vi "ArmGoToPosition.vi"(0 "RobotConfig":T15={"Motors"={"DriveRightPrimary"={"CAN Address"=3, "Invert"=FALSE, "InvertSensor"=FALSE, "Unit Conversion Factor"=0.0, "Brake Mode"=enum."Override to Brake", "Reverse Limt Switch Mode"=enum."Normally Closed", "Forward Limt Swith Mode"=enum."Normally Closed", "PWM Channel"=enum."Invalid", "Motor Controller Type"=enum."Talon SRX", "Peak Current (A)"=0, "Continuous Current (A)"=0, "Peak Duration (ms)"=0, "Current Limit Enable"=FALSE}, "DriveRightSecondary"={"CAN Address"=2, "Invert"=FALSE, "InvertSensor"=FALSE, "Unit Conversion Factor"=0.0, "Brake Mode"=enum."Override to Brake", "Reverse Limt Switch Mode"=enum."Normally Closed", "Forward Limt Swith Mode"=enum."Normally Closed", "PWM Channel"=enum."Invalid", "Motor Controller Type"=enum."Talon SRX", "Peak Current (A)"=0, "Continuous Current (A)"=0, "Peak Duration (ms)"=0, "Current Limit Enable"=FALSE}, "DriveLeftPrimary"={"CAN Address"=1, "Invert"=FALSE, "InvertSensor"=FALSE, "Unit Conversion Factor"=0.0, "Brake Mode"=enum."Override to Brake", "Reverse Limt Switch Mode"=enum."Normally Closed", "Forward Limt Swith Mode"=enum."Normally Closed", "PWM Channel"=enum."Invalid", "Motor Controller Type"=enum."Talon SRX", "Peak Current (A)"=0, "Continuous Current (A)"=0, "Peak Duration (ms)"=0, "Current Limit Enable"=FALSE}, "DriveLeftSecondary"={"CAN Address"=4, "Invert"=FALSE, "InvertSensor"=FALSE, "Unit Conversion Factor"=0.0, "Brake Mode"=enum."Override to Brake", "Reverse Limt Switch Mode"=enum."Normally Closed", "Forward Limt Swith Mode"=enum."Normally Closed", "PWM Channel"=enum."Invalid", "Motor Controller Type"=enum."Talon SRX", "Peak Current (A)"=0, "Continuous Current (A)"=0, "Peak Duration (ms)"=0, "Current Limit Enable"=FALSE}, "RearClimb"={"CAN Address"=8, "Invert"=FALSE, "InvertSensor"=FALSE, "Unit Conversion Factor"=0.0, "Brake Mode"=enum."Override to Brake", "Reverse Limt Switch Mode"=enum."Normally Closed", "Forward Limt Swith Mode"=enum."Normally Closed", "PWM Channel"=enum."Invalid", "Motor Controller Type"=enum."Talon SRX", "Peak Current (A)"=0, "Continuous Current (A)"=0, "Peak Duration (ms)"=0, "Current Limit Enable"=FALSE}, "Front Climb"={"CAN Address"=7, "Invert"=FALSE, "InvertSensor"=FALSE, "Unit Conversion Factor"=0.0, "Brake Mode"=enum."Override to Brake", "Reverse Limt Switch Mode"=enum."Normally Closed", "Forward Limt Swith Mode"=enum."Normally Closed", "PWM Channel"=enum."Invalid", "Motor Controller Type"=enum."Talon SRX", "Peak Current (A)"=0, "Continuous Current (A)"=0, "Peak Duration (ms)"=0, "Current Limit Enable"=FALSE}, "Climb Drive"={"CAN Address"=5, "Invert"=FALSE, "InvertSensor"=FALSE, "Unit Conversion Factor"=0.0, "Brake Mode"=enum."Override to Brake", "Reverse Limt Switch Mode"=enum."Normally Closed", "Forward Limt Swith Mode"=enum."Normally Closed", "PWM Channel"=enum."Invalid", "Motor Controller Type"=enum."Talon SRX", "Peak Current (A)"=0, "Continuous Current (A)"=0, "Peak Duration (ms)"=0, "Current Limit Enable"=FALSE}, "Shoulder1"={"CAN Address"=6, "Invert"=FALSE, "InvertSensor"=FALSE, "Unit Conversion Factor"=0.0, "Brake Mode"=enum."Override to Brake", "Reverse Limt Switch Mode"=enum."Normally Closed", "Forward Limt Swith Mode"=enum."Normally Closed", "PWM Channel"=enum."Invalid", "Motor Controller Type"=enum."Talon SRX", "Peak Current (A)"=0, "Continuous Current (A)"=0, "Peak Duration (ms)"=0, "Current Limit Enable"=FALSE}, "Shoulder2"={"CAN Address"=9, "Invert"=FALSE, "InvertSensor"=FALSE, "Unit Conversion Factor"=0.0, "Brake Mode"=enum."Override to Brake", "Reverse Limt Switch Mode"=enum."Normally Closed", "Forward Limt Swith Mode"=enum."Normally Closed", "PWM Channel"=enum."Invalid", "Motor Controller Type"=enum."Talon SRX", "Peak Current (A)"=0, "Continuous Current (A)"=0, "Peak Duration (ms)"=0, "Current Limit Enable"=FALSE}, "Wrist"={"CAN Address"=10, "Invert"=FALSE, "InvertSensor"=FALSE, "Unit Conversion Factor"=0.0, "Brake Mode"=enum."Override to Brake", "Reverse Limt Switch Mode"=enum."Disabled", "Forward Limt Swith Mode"=enum."Disabled", "PWM Channel"=enum."Invalid", "Motor Controller Type"=enum."Talon SRX", "Peak Current (A)"=0, "Continuous Current (A)"=0, "Peak Duration (ms)"=0, "Current Limit Enable"=FALSE}, "Extension"={"CAN Address"=11, "Invert"=FALSE, "InvertSensor"=FALSE, "Unit Conversion Factor"=0.0, "Brake Mode"=enum."Override to Brake", "Reverse Limt Switch Mode"=enum."Disabled", "Forward Limt Swith Mode"=enum."Disabled", "PWM Channel"=enum."Invalid", "Motor Controller Type"=enum."Talon SRX", "Peak Current (A)"=0, "Continuous Current (A)"=0, "Peak Duration (ms)"=0, "Current Limit Enable"=FALSE}, "CargoIntake"={"CAN Address"=0, "Invert"=FALSE, "InvertSensor"=FALSE, "Unit Conversion Factor"=1.0, "Brake Mode"=enum."Override to Brake", "Reverse Limt Switch Mode"=enum."Disabled", "Forward Limt Swith Mode"=enum."Normally Open", "PWM Channel"=enum."PWM 8", "Motor Controller Type"=enum."Talon SR", "Peak Current (A)"=0, "Continuous Current (A)"=0, "Peak Duration (ms)"=0, "Current Limit Enable"=FALSE}, "Intake2"={"CAN Address"=10, "Invert"=FALSE, "InvertSensor"=TRUE, "Unit Conversion Factor"=0.0, "Brake Mode"=enum."Override to Brake", "Reverse Limt Switch Mode"=enum."Normally Open", "Forward Limt Swith Mode"=enum."Normally Open", "PWM Channel"=enum."PWM 0", "Motor Controller Type"=enum."Disabled", "Peak Current (A)"=0, "Continuous Current (A)"=0, "Peak Duration (ms)"=0, "Current Limit Enable"=FALSE}}, "Sensors"={"IMU"={"Yaw Axis"=enum."Z", "SPI Bus"=enum."SPI MXP", "AHRS Algorithm"=enum."Complementary", "Calibration Time (s)"=3.0, "Calibrate On Open"=TRUE}, "HomingButton"={"DIOChannel"=enum."DIO 0", "Active Low"=FALSE}, "HomingLED_Green"={"DIOChannel"=enum."DIO 0", "Active Low"=FALSE}, "HomingLED_Yellow"={"DIOChannel"=enum."DIO 0", "Active Low"=FALSE}, "HomingLED_Red"={"DIOChannel"=enum."DIO 0", "Active Low"=FALSE}}, "PID"={"FrontClimb"={"P"=0.0, "I"=0.0, "D"=0.0, "F"=0.0, "IZone"=0.0}, "RearClimb"={"P"=0.0, "I"=0.0, "D"=0.0, "F"=0.0, "IZone"=0.0}, "ArmShoulder"={"P"=0.0, "I"=0.0, "D"=0.0, "F"=0.0, "IZone"=0.0}, "ArmExtend"={"P"=0.0, "I"=0.0, "D"=0.0, "F"=0.0, "IZone"=0.0}, "ArmWrist"={"P"=0.0, "I"=0.0, "D"=0.0, "F"=0.0, "IZone"=0.0}}, "Solenoids"={" Shifter"={"SolenoidChannel"=enum."Solenoid 3", "Invert"=FALSE}, "Hatch Grip"={"SolenoidChannel"=enum."Solenoid 0", "Invert"=FALSE}, "Hatch Extend"={"SolenoidChannel"=enum."Solenoid 1", "Invert"=FALSE}, "Manipulator Slide"={"SolenoidChannel"=enum."Solenoid 2", "Invert"=FALSE}, "Hatch Floor Intake"={"SolenoidChannel"=enum."Solenoid 0", "Invert"=FALSE}}, "Enable Compressor"=TRUE, "MotionMagic"={"FrontClimbExtend"={"CruiseVelocity"=0, "Acceleration"=0}, "RearClimbExtend"={"CruiseVelocity"=0, "Acceleration"=0}, "FrontClimbRetract"={"CruiseVelocity"=0, "Acceleration"=0}, "RearClimbRetract"={"CruiseVelocity"=0, "Acceleration"=0}}, "RobotDimensions"={"Length (in)"=0.0, "Shoulder Height (in)"=0.0, "Frame Height (in)"=0.0, "Arm Center to Front of Robot (in)"=0.0, "Arm Min Extension (in)"=0.0, "Arm Max Extension (in)"=0.0, "Cargo Intake Loop Length (in)"=0.0, "Cargo Intake Loop Width (in)"=0.0, "Cargo Intake Loop Offset (in)"=0.0, "Cargo Intake Loop Angle (rad)"=0.0}, "Arm Home Position"={"Radius (in)"=0.0, "ShoulderAngle (rad)"=0.0, "WristAngle (rad)"=0.0}, "Climb Home Position"={"Back Climb"=0.0, "Front Climb"=0.0}, "Climb Positions"={"Retract"=0.0, "Level 2"=0.0, "Level 3"=0.0}}, 1 "ArmPlanRequest":T10={"Destination"=enum."Forward Cargo Feeder Station", "Preview"=FALSE, "Start"=enum."Forward Cargo Feeder Station", "Fixed Start"=FALSE}, 2 "Arm min Extension (in)":dbl, 3 "Arm max Extension (in)":dbl, 4 "Game Piece Position":T32, 5 "Avoidance Polygon":T30, 6 "RobotMotors":T4={"DriveRightPrimary"={"DeviceStatus"={"status"=FALSE, "code"=0, "source"=""}, "Type"=enum."PWM", "PWM"={"PWM Channel"=enum."PWM 1", "DeadBand"={"Name"="", "maxPositivePwm"=0, "minPositivePwm"=0, "centerPwm"=0, "maxNegativePwm"=0, "minNegativePwm"=0, "angularRange"=0}}, "CAN"={"Device Number"=0, "SetOutput VI Ref"=variant(enum8{"Percent VBus", "Current", "Speed", "Position", "Voltage"} enum."Percent VBus"), "GetOutput VI Ref"=variant(refnum<k1> refnum), "Enable VI Ref"=variant(dbl 12.0), "Disable VI Ref"=variant(enum8{"Percent VBus", "Speed", "Position", "Slave", "Unchanged / Invalid", "Voltage Compensation", "Current", "Motion Profile"} enum."Percent VBus"), "Data"=variant}, "Invert"=FALSE, "DIO PWM"={"PWM \"Enable\" Channel"=enum."Invalid", "DIOChannel"=enum."Invalid", "PWM Rate"=0.0}}, "DriveRightSecondary"={"DeviceStatus"={"status"=FALSE, "code"=0, "source"=""}, "Type"=enum."PWM", "PWM"={"PWM Channel"=enum."PWM 1", "DeadBand"={"Name"="", "maxPositivePwm"=0, "minPositivePwm"=0, "centerPwm"=0, "maxNegativePwm"=0, "minNegativePwm"=0, "angularRange"=0}}, "CAN"={"Device Number"=0, "SetOutput VI Ref"=variant(enum8{"Percent VBus", "Current", "Speed", "Position", "Voltage"} enum."Percent VBus"), "GetOutput VI Ref"=variant(refnum<k1> refnum), "Enable VI Ref"=variant(dbl 12.0), "Disable VI Ref"=variant(enum8{"Percent VBus", "Speed", "Position", "Slave", "Unchanged / Invalid", "Voltage Compensation", "Current", "Motion Profile"} enum."Percent VBus"), "Data"=variant}, "Invert"=FALSE, "DIO PWM"={"PWM \"Enable\" Channel"=enum."Invalid", "DIOChannel"=enum."Invalid", "PWM Rate"=0.0}}, "DriveLeftPrimary"={"DeviceStatus"={"status"=FALSE, "code"=0, "source"=""}, "Type"=enum."PWM", "PWM"={"PWM Channel"=enum."PWM 1", "DeadBand"={"Name"="", "maxPositivePwm"=0, "minPositivePwm"=0, "centerPwm"=0, "maxNegativePwm"=0, "minNegativePwm"=0, "angularRange"=0}}, "CAN"={"Device Number"=0, "SetOutput VI Ref"=variant(enum8{"Percent VBus", "Current", "Speed", "Position", "Voltage"} enum."Percent VBus"), "GetOutput VI Ref"=variant(refnum<k1> refnum), "Enable VI Ref"=variant(dbl 12.0), "Disable VI Ref"=variant(enum8{"Percent VBus", "Speed", "Position", "Slave", "Unchanged / Invalid", "Voltage Compensation", "Current", "Motion Profile"} enum."Percent VBus"), "Data"=variant}, "Invert"=FALSE, "DIO PWM"={"PWM \"Enable\" Channel"=enum."Invalid", "DIOChannel"=enum."Invalid", "PWM Rate"=0.0}}, "DriveLeftSecondary"={"DeviceStatus"={"status"=FALSE, "code"=0, "source"=""}, "Type"=enum."PWM", "PWM"={"PWM Channel"=enum."PWM 1", "DeadBand"={"Name"="", "maxPositivePwm"=0, "minPositivePwm"=0, "centerPwm"=0, "maxNegativePwm"=0, "minNegativePwm"=0, "angularRange"=0}}, "CAN"={"Device Number"=0, "SetOutput VI Ref"=variant(enum8{"Percent VBus", "Current", "Speed", "Position", "Voltage"} enum."Percent VBus"), "GetOutput VI Ref"=variant(refnum<k1> refnum), "Enable VI Ref"=variant(dbl 12.0), "Disable VI Ref"=variant(enum8{"Percent VBus", "Speed", "Position", "Slave", "Unchanged / Invalid", "Voltage Compensation", "Current", "Motion Profile"} enum."Percent VBus"), "Data"=variant}, "Invert"=FALSE, "DIO PWM"={"PWM \"Enable\" Channel"=enum."Invalid", "DIOChannel"=enum."Invalid", "PWM Rate"=0.0}}, " RearClimb"={"DeviceStatus"={"status"=FALSE, "code"=0, "source"=""}, "Type"=enum."PWM", "PWM"={"PWM Channel"=enum."PWM 1", "DeadBand"={"Name"="", "maxPositivePwm"=0, "minPositivePwm"=0, "centerPwm"=0, "maxNegativePwm"=0, "minNegativePwm"=0, "angularRange"=0}}, "CAN"={"Device Number"=0, "SetOutput VI Ref"=variant(enum8{"Percent VBus", "Current", "Speed", "Position", "Voltage"} enum."Percent VBus"), "GetOutput VI Ref"=variant(refnum<k1> refnum), "Enable VI Ref"=variant(dbl 12.0), "Disable VI Ref"=variant(enum8{"Percent VBus", "Speed", "Position", "Slave", "Unchanged / Invalid", "Voltage Compensation", "Current", "Motion Profile"} enum."Percent VBus"), "Data"=variant}, "Invert"=FALSE, "DIO PWM"={"PWM \"Enable\" Channel"=enum."Invalid", "DIOChannel"=enum."Invalid", "PWM Rate"=0.0}}, "FrontClimb"={"DeviceStatus"={"status"=FALSE, "code"=0, "source"=""}, "Type"=enum."PWM", "PWM"={"PWM Channel"=enum."PWM 1", "DeadBand"={"Name"="", "maxPositivePwm"=0, "minPositivePwm"=0, "centerPwm"=0, "maxNegativePwm"=0, "minNegativePwm"=0, "angularRange"=0}}, "CAN"={"Device Number"=0, "SetOutput VI Ref"=variant(enum8{"Percent VBus", "Current", "Speed", "Position", "Voltage"} enum."Percent VBus"), "GetOutput VI Ref"=variant(refnum<k1> refnum), "Enable VI Ref"=variant(dbl 12.0), "Disable VI Ref"=variant(enum8{"Percent VBus", "Speed", "Position", "Slave", "Unchanged / Invalid", "Voltage Compensation", "Current", "Motion Profile"} enum."Percent VBus"), "Data"=variant}, "Invert"=FALSE, "DIO PWM"={"PWM \"Enable\" Channel"=enum."Invalid", "DIOChannel"=enum."Invalid", "PWM Rate"=0.0}}, "ClimbDrive"={"DeviceStatus"={"status"=FALSE, "code"=0, "source"=""}, "Type"=enum."PWM", "PWM"={"PWM Channel"=enum."PWM 1", "DeadBand"={"Name"="", "maxPositivePwm"=0, "minPositivePwm"=0, "centerPwm"=0, "maxNegativePwm"=0, "minNegativePwm"=0, "angularRange"=0}}, "CAN"={"Device Number"=0, "SetOutput VI Ref"=variant(enum8{"Percent VBus", "Current", "Speed", "Position", "Voltage"} enum."Percent VBus"), "GetOutput VI Ref"=variant(refnum<k1> refnum), "Enable VI Ref"=variant(dbl 12.0), "Disable VI Ref"=variant(enum8{"Percent VBus", "Speed", "Position", "Slave", "Unchanged / Invalid", "Voltage Compensation", "Current", "Motion Profile"} enum."Percent VBus"), "Data"=variant}, "Invert"=FALSE, "DIO PWM"={"PWM \"Enable\" Channel"=enum."Invalid", "DIOChannel"=enum."Invalid", "PWM Rate"=0.0}}, "Shoulder2"={"DeviceStatus"={"status"=FALSE, "code"=0, "source"=""}, "Type"=enum."PWM", "PWM"={"PWM Channel"=enum."PWM 1", "DeadBand"={"Name"="", "maxPositivePwm"=0, "minPositivePwm"=0, "centerPwm"=0, "maxNegativePwm"=0, "minNegativePwm"=0, "angularRange"=0}}, "CAN"={"Device Number"=0, "SetOutput VI Ref"=variant(enum8{"Percent VBus", "Current", "Speed", "Position", "Voltage"} enum."Percent VBus"), "GetOutput VI Ref"=variant(refnum<k1> refnum), "Enable VI Ref"=variant(dbl 12.0), "Disable VI Ref"=variant(enum8{"Percent VBus", "Speed", "Position", "Slave", "Unchanged / Invalid", "Voltage Compensation", "Current", "Motion Profile"} enum."Percent VBus"), "Data"=variant}, "Invert"=FALSE, "DIO PWM"={"PWM \"Enable\" Channel"=enum."Invalid", "DIOChannel"=enum."Invalid", "PWM Rate"=0.0}}, "Shoulder1 "={"DeviceStatus"={"status"=FALSE, "code"=0, "source"=""}, "Type"=enum."PWM", "PWM"={"PWM Channel"=enum."PWM 1", "DeadBand"={"Name"="", "maxPositivePwm"=0, "minPositivePwm"=0, "centerPwm"=0, "maxNegativePwm"=0, "minNegativePwm"=0, "angularRange"=0}}, "CAN"={"Device Number"=0, "SetOutput VI Ref"=variant(enum8{"Percent VBus", "Current", "Speed", "Position", "Voltage"} enum."Percent VBus"), "GetOutput VI Ref"=variant(refnum<k1> refnum), "Enable VI Ref"=variant(dbl 12.0), "Disable VI Ref"=variant(enum8{"Percent VBus", "Speed", "Position", "Slave", "Unchanged / Invalid", "Voltage Compensation", "Current", "Motion Profile"} enum."Percent VBus"), "Data"=variant}, "Invert"=FALSE, "DIO PWM"={"PWM \"Enable\" Channel"=enum."Invalid", "DIOChannel"=enum."Invalid", "PWM Rate"=0.0}}, "Wrist"={"DeviceStatus"={"status"=FALSE, "code"=0, "source"=""}, "Type"=enum."PWM", "PWM"={"PWM Channel"=enum."PWM 1", "DeadBand"={"Name"="", "maxPositivePwm"=0, "minPositivePwm"=0, "centerPwm"=0, "maxNegativePwm"=0, "minNegativePwm"=0, "angularRange"=0}}, "CAN"={"Device Number"=0, "SetOutput VI Ref"=variant(enum8{"Percent VBus", "Current", "Speed", "Position", "Voltage"} enum."Percent VBus"), "GetOutput VI Ref"=variant(refnum<k1> refnum), "Enable VI Ref"=variant(dbl 12.0), "Disable VI Ref"=variant(enum8{"Percent VBus", "Speed", "Position", "Slave", "Unchanged / Invalid", "Voltage Compensation", "Current", "Motion Profile"} enum."Percent VBus"), "Data"=variant}, "Invert"=FALSE, "DIO PWM"={"PWM \"Enable\" Channel"=enum."Invalid", "DIOChannel"=enum."Invalid", "PWM Rate"=0.0}}, "Extension"={"DeviceStatus"={"status"=FALSE, "code"=0, "source"=""}, "Type"=enum."PWM", "PWM"={"PWM Channel"=enum."PWM 1", "DeadBand"={"Name"="", "maxPositivePwm"=0, "minPositivePwm"=0, "centerPwm"=0, "maxNegativePwm"=0, "minNegativePwm"=0, "angularRange"=0}}, "CAN"={"Device Number"=0, "SetOutput VI Ref"=variant(enum8{"Percent VBus", "Current", "Speed", "Position", "Voltage"} enum."Percent VBus"), "GetOutput VI Ref"=variant(refnum<k1> refnum), "Enable VI Ref"=variant(dbl 12.0), "Disable VI Ref"=variant(enum8{"Percent VBus", "Speed", "Position", "Slave", "Unchanged / Invalid", "Voltage Compensation", "Current", "Motion Profile"} enum."Percent VBus"), "Data"=variant}, "Invert"=FALSE, "DIO PWM"={"PWM \"Enable\" Channel"=enum."Invalid", "DIOChannel"=enum."Invalid", "PWM Rate"=0.0}}, "CargoIntake"={"DeviceStatus"={"status"=FALSE, "code"=0, "source"=""}, "Type"=enum."PWM", "PWM"={"PWM Channel"=enum."PWM 1", "DeadBand"={"Name"="", "maxPositivePwm"=0, "minPositivePwm"=0, "centerPwm"=0, "maxNegativePwm"=0, "minNegativePwm"=0, "angularRange"=0}}, "CAN"={"Device Number"=0, "SetOutput VI Ref"=variant(enum8{"Percent VBus", "Current", "Speed", "Position", "Voltage"} enum."Percent VBus"), "GetOutput VI Ref"=variant(refnum<k1> refnum), "Enable VI Ref"=variant(dbl 12.0), "Disable VI Ref"=variant(enum8{"Percent VBus", "Speed", "Position", "Slave", "Unchanged / Invalid", "Voltage Compensation", "Current", "Motion Profile"} enum."Percent VBus"), "Data"=variant}, "Invert"=FALSE, "DIO PWM"={"PWM \"Enable\" Channel"=enum."Invalid", "DIOChannel"=enum."Invalid", "PWM Rate"=0.0}}, "Intake2"={"DeviceStatus"={"status"=FALSE, "code"=0, "source"=""}, "Type"=enum."PWM", "PWM"={"PWM Channel"=enum."PWM 1", "DeadBand"={"Name"="", "maxPositivePwm"=0, "minPositivePwm"=0, "centerPwm"=0, "maxNegativePwm"=0, "minNegativePwm"=0, "angularRange"=0}}, "CAN"={"Device Number"=0, "SetOutput VI Ref"=variant(enum8{"Percent VBus", "Current", "Speed", "Position", "Voltage"} enum."Percent VBus"), "GetOutput VI Ref"=variant(refnum<k1> refnum), "Enable VI Ref"=variant(dbl 12.0), "Disable VI Ref"=variant(enum8{"Percent VBus", "Speed", "Position", "Slave", "Unchanged / Invalid", "Voltage Compensation", "Current", "Motion Profile"} enum."Percent VBus"), "Data"=variant}, "Invert"=FALSE, "DIO PWM"={"PWM \"Enable\" Channel"=enum."Invalid", "DIOChannel"=enum."Invalid", "PWM Rate"=0.0}}}, 7 "MotionProfileGeneratorParameters":T29={"Trajectory Point Interval (ms)"=10, "Maximum Travel Speed (units/s)"=0.0, "Velocity Ramp Time (ms)"=0.0, "Acceleration Ramp Time (ms)"=1.0} {"Acceleration Ramp Time (ms)" min=1.0; "Velocity Ramp Time (ms)" min=1.0; "Maximum Travel Speed (units/s)" min=0.0; "Trajectory Point Interval (ms)" items=["TrajectoryDuration_0ms"=0, "TrajectoryDuration_5ms"=5, "TrajectoryDuration_10ms"=10, "TrajectoryDuration_20ms"=20, "TrajectoryDuration_30ms"=30, "TrajectoryDuration_40ms"=40, "TrajectoryDuration_50ms"=50, "TrajectoryDuration_100ms"=100]}, 8 "Arm Pass Through Params":T2, 9 "RobotDimensions":T3, 10 "TestMode":bool, 11 "Test_ArmAbsolutePose":T1) -> (14 "ArmPlanResponse":T12 {"WristTrajectory"."Time (ms)" items=["TrajectoryDuration_0ms"=0, "TrajectoryDuration_5ms"=5, "TrajectoryDuration_10ms"=10, "TrajectoryDuration_20ms"=20, "TrajectoryDuration_30ms"=30, "TrajectoryDuration_40ms"=40, "TrajectoryDuration_50ms"=50, "TrajectoryDuration_100ms"=100]; "ExtendTrajectory"."Time (ms)" items=["TrajectoryDuration_0ms"=0, "TrajectoryDuration_5ms"=5, "TrajectoryDuration_10ms"=10, "TrajectoryDuration_20ms"=20, "TrajectoryDuration_30ms"=30, "TrajectoryDuration_40ms"=40, "TrajectoryDuration_50ms"=50, "TrajectoryDuration_100ms"=100]; "ShoulderTrajectory"."Time (ms)" items=["TrajectoryDuration_0ms"=0, "TrajectoryDuration_5ms"=5, "TrajectoryDuration_10ms"=10, "TrajectoryDuration_20ms"=20, "TrajectoryDuration_30ms"=30, "TrajectoryDuration_40ms"=40, "TrajectoryDuration_50ms"=50, "TrajectoryDuration_100ms"=100]})   [LabVIEW 2018]
uses:
  TypeDefs/GamePiecePosition.ctl
  TypeDefs/ArmPositions.ctl
  TypeDefs/ArmAbsolutePosition.ctl
  ArgosLib/Path Planning/TypeDefs/Polygon2D.ctl
  ArgosLib/Path Planning/TypeDefs/Point2D.ctl
  ArgosLib/MotionProfiling/TypeDefs/MotionProfileGeneratorParams.ctl
  <vilib>/Rock Robotics/WPI/ThirdParty/Phoenix-LabVIEW/Motor Controller/Controls/CTRE_Phoenix_MotorControl_TrajectoryPointTimeDur.ctl
  TypeDefs/ConfigComponents/Config_Robot.ctl
  ArgosLib/Config/ConfigComponents/TypeDefs/Config_Motor.ctl
  <vilib>/Rock Robotics/WPI/ThirdParty/Phoenix-LabVIEW/Motor Controller/Controls/CTRE_Phoenix_MotorControl_NeutralMode.ctl
  <vilib>/Rock Robotics/WPI/ThirdParty/Phoenix-LabVIEW/Motor Controller/Controls/CTRE_Phoenix_MotorControl_LimitSwitchNormal.ctl
  <vilib>/Rock Robotics/SystemInterfaces/DIO/FPGA_DIOPWMChannel.ctl
  ArgosLib/Config/ConfigComponents/TypeDefs/Config_MotorCtrlType.ctl
  ArgosLib/Config/ConfigComponents/TypeDefs/Config_IMU.ctl
  <vilib>/Rock Robotics/SystemInterfaces/spilib/spi_bus.ctl
  ArgosLib/Config/ConfigComponents/TypeDefs/Config_DigitalIO.ctl
  <vilib>/Rock Robotics/SystemInterfaces/DIO/FPGA_DIOChannel.ctl
  ArgosLib/Config/ConfigComponents/TypeDefs/Config_PIDParams.ctl
  ArgosLib/Config/ConfigComponents/TypeDefs/Config_SingleSolenoid.ctl
  <vilib>/Rock Robotics/WPI/Solenoid/WPI_SolenoidChannel.ctl
  ArgosLib/Config/ConfigComponents/TypeDefs/Config_MotionMagicParams.ctl
  TypeDefs/ConfigComponents/Config_Dimensions.ctl
  TypeDefs/ArmCoordinate.ctl
  Climber/TypeDefs/ClimberPositionHeights.ctl
  TypeDefs/ArmPlanResponse.ctl
  ArgosLib/MotionProfiling/TypeDefs/TrajectoryPoint.ctl
  TypeDefs/ArmPlanRequest.ctl
  TypeDefs/ArmTargetPosition.ctl
  TypeDefs/RobotComponents/RobotMotors.ctl
  <vilib>/Rock Robotics/WPI/MotorControl/WPI_MotorControlDeviceRef.ctl
  <vilib>/Rock Robotics/WPI/MotorControl/WPI_MotorControlType.ctl
  <vilib>/Rock Robotics/WPI/PWM/WPI_PWMDeadband.ctl
  TypeDefs/ArmPassThroughParams.ctl
  <vilib>/Playing With Fusion Inc/Playing With Fusion Lib for FRC/PWF_Venom_LabVIEW/Public/PwF_Venom_GetPosition.vi
  <vilib>/Rock Robotics/WPI/ThirdParty/Phoenix-LabVIEW/Motor Controller/Get/CTRE_Phoenix_MotorController_GetSelectedSensorData.vi
  ArgosLib/ArgosLib.lvlib
  <vilib>/Playing With Fusion Inc/Playing With Fusion Lib for FRC/PWF_Venom_LabVIEW/PwF_Venom.lvlib
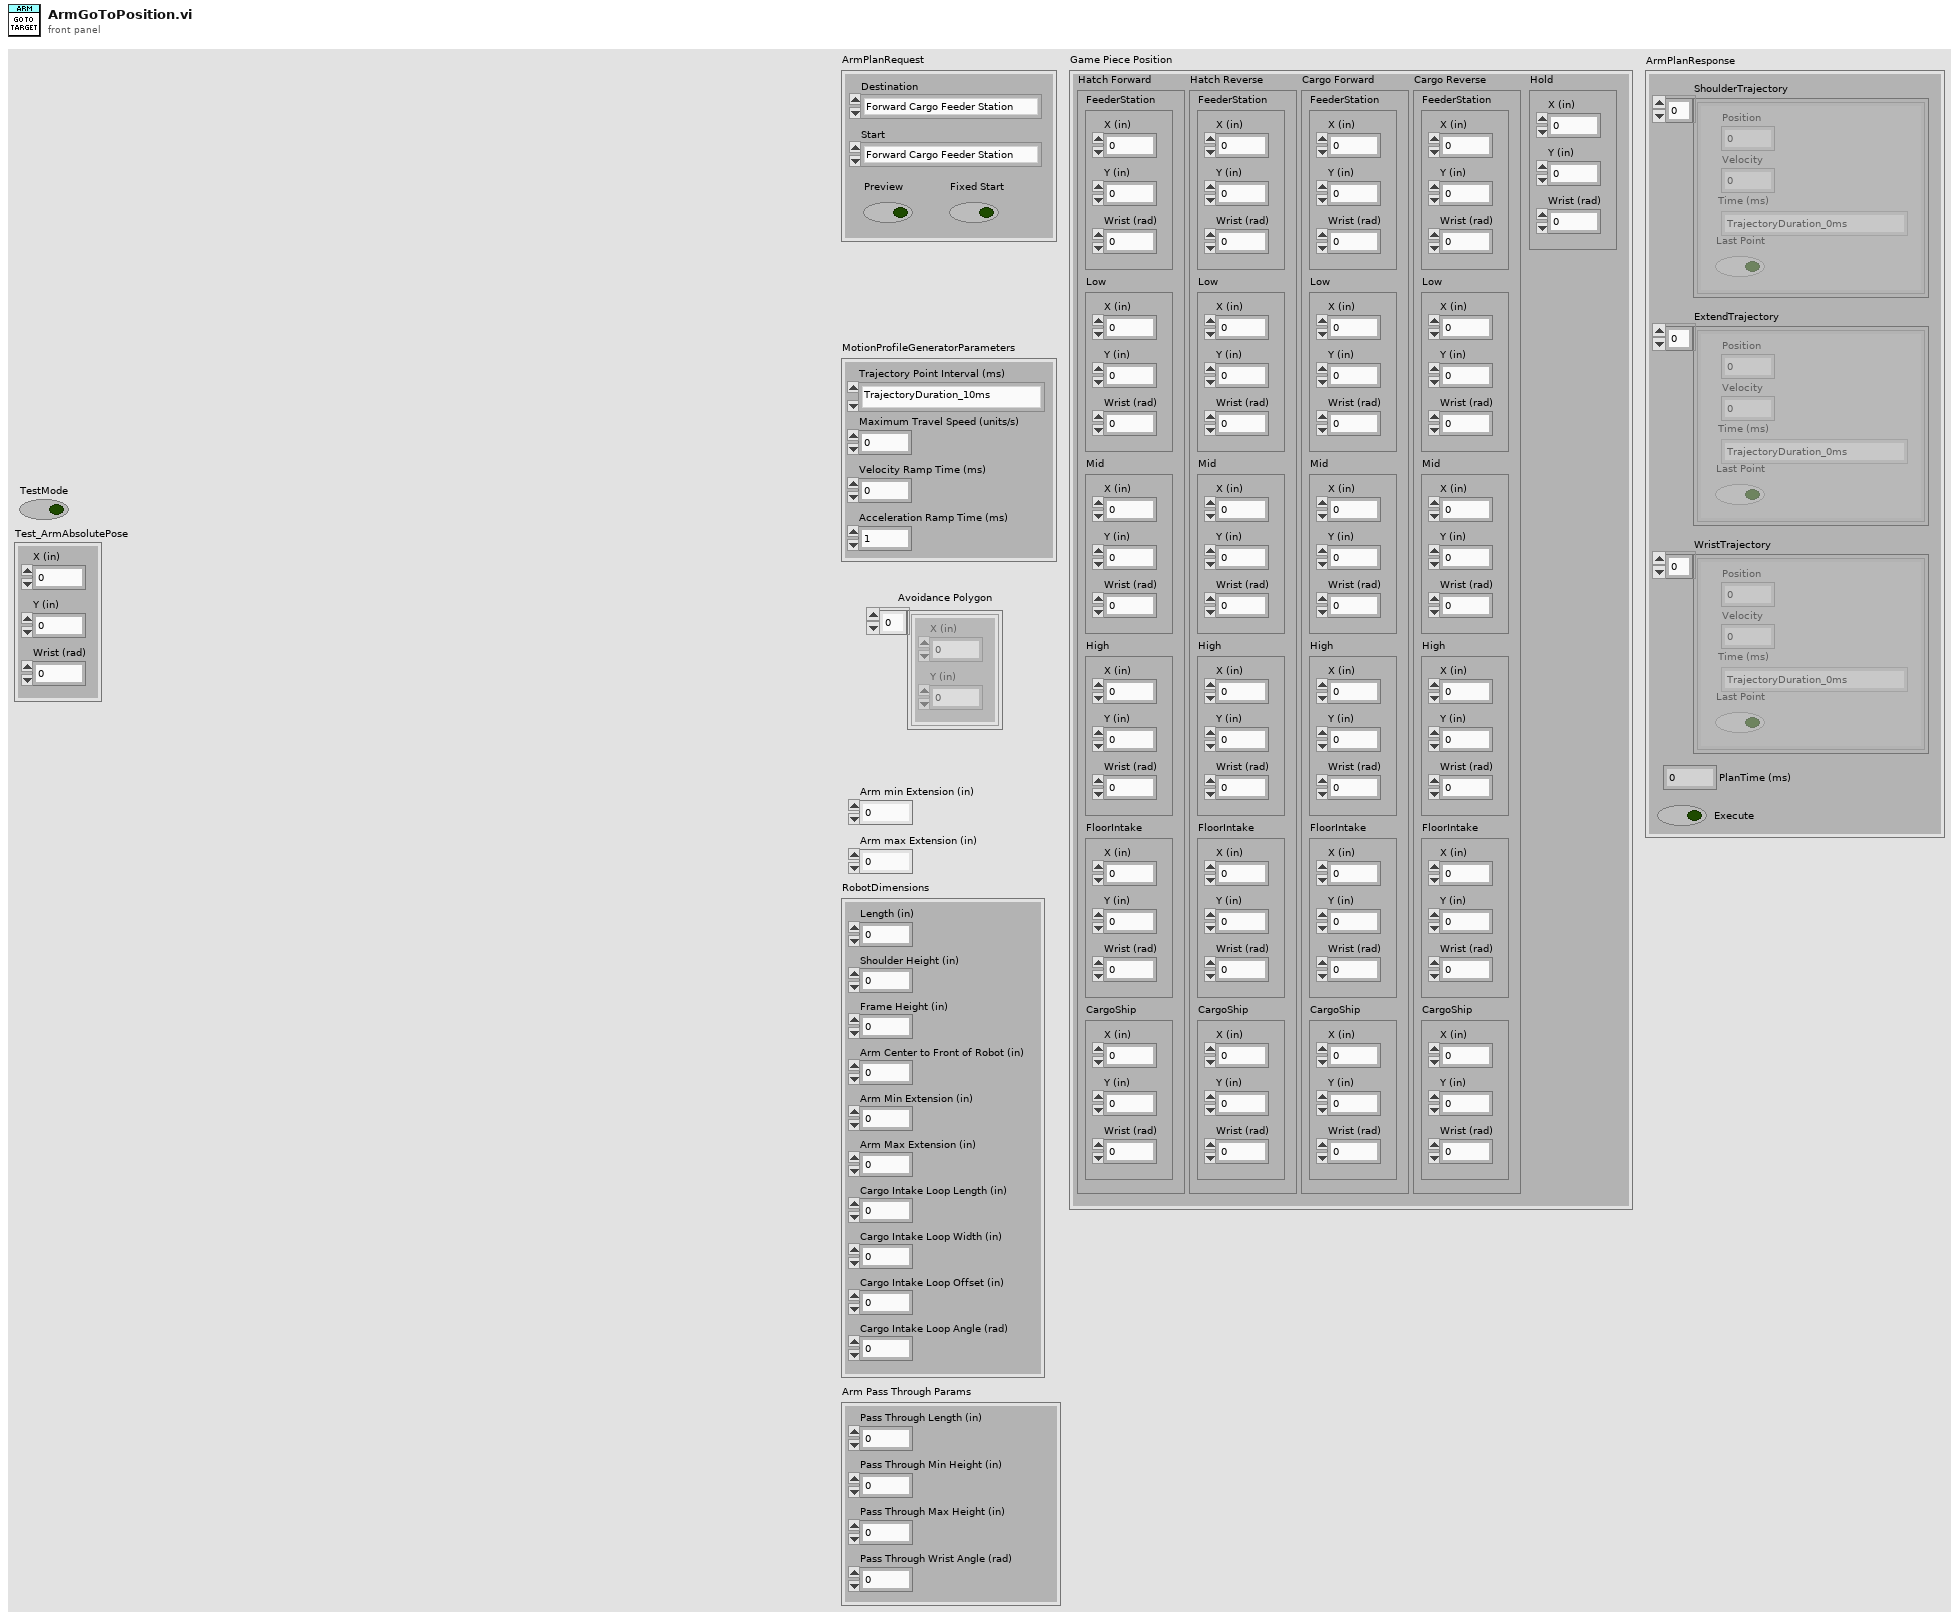
[diagram p1: front panel]
types:
  T1 = typedef "ArmAbsolutePosition.ctl" = cluster{"X (in)":dbl, "Y (in)":dbl, "Wrist (rad)":dbl}
  T2 = typedef "ArmPassThroughParams.ctl" = cluster{"Pass Through Length (in)":dbl, "Pass Through Min Height (in)":dbl, "Pass Through Max Height (in)":dbl, "Pass Through Wrist Angle (rad)":dbl}
  T3 = typedef "Config_Dimensions.ctl" = cluster{"Length (in)":dbl, "Shoulder Height (in)":dbl, "Frame Height (in)":dbl, "Arm Center to Front of Robot (in)":dbl, "Arm Min Extension (in)":dbl, "Arm Max Extension (in)":dbl, "Cargo Intake Loop Length (in)":dbl, "Cargo Intake Loop Width (in)":dbl, "Cargo Intake Loop Offset (in)":dbl, "Cargo Intake Loop Angle (rad)":dbl}
  T4 = typedef "RobotMotors.ctl" = cluster{"DriveRightPrimary":T5, "DriveRightSecondary":T5, "DriveLeftPrimary":T5, "DriveLeftSecondary":T5, " RearClimb":T5, "FrontClimb":T5, "ClimbDrive":T5, "Shoulder2":T5, "Shoulder1 ":T5, "Wrist":T5, "Extension":T5, "CargoIntake":T5, "Intake2":T5}
  T5 = typedef "WPI_MotorControlDeviceRef.ctl" = cluster{"DeviceStatus":errorcluster, "Type":T6, "PWM":cluster{"PWM Channel":T7, "DeadBand":T8}, "CAN":cluster{"Device Number":u8, "SetOutput VI Ref":variant, "GetOutput VI Ref":variant, "Enable VI Ref":variant, "Disable VI Ref":variant, "Data":variant}, "Invert":bool, "DIO PWM":cluster{"PWM \"Enable\" Channel":T7, "DIOChannel":T9, "PWM Rate":dbl}}
  T6 = typedef "WPI_MotorControlType.ctl" = enum16{"PWM", "CAN", "DIO PWM"}
  T7 = typedef "FPGA_DIOPWMChannel.ctl" = enum8{"PWM 0", "PWM 1", "PWM 2", "PWM 3", "PWM 4", "PWM 5", "PWM 6", "PWM 7", "PWM 8", "PWM 9", "PWM MXP 0", "PWM MXP 1", "PWM MXP 2", "PWM MXP 3", "PWM MXP 4", "PWM MXP 5", "PWM MXP 6", "PWM MXP 7", "PWM MXP 8", "PWM MXP 9", "Invalid"}
  T8 = typedef "WPI_PWMDeadband.ctl" = cluster{"Name":string, "maxPositivePwm":i32, "minPositivePwm":i32, "centerPwm":i32, "maxNegativePwm":i32, "minNegativePwm":i32, "angularRange":u16}
  T9 = typedef "FPGA_DIOChannel.ctl" = enum8{"DIO 0", "DIO 1", "DIO 2", "DIO 3", "DIO 4", "DIO 5", "DIO 6", "DIO 7", "DIO 8", "DIO 9", "DIO MXP 0", "DIO MXP 1", "DIO MXP 2", "DIO MXP 3", "DIO MXP 4", "DIO MXP 5", "DIO MXP 6", "DIO MXP 7", "DIO MXP 8", "DIO MXP 9", "DIO MXP 10", "DIO MXP 11", "DIO MXP 12", "DIO MXP 13", "DIO MXP 14", "DIO MXP 15", "SPI Port CS1", "SPI Port CS2", "SPI Port CS3", "SPI Port MISO", "SPI Port MOSI", "Invalid"}
  T10 = typedef "ArmPlanRequest.ctl" = cluster{"Destination":T11, "Preview":bool, "Start":T11, "Fixed Start":bool}
  T11 = typedef "ArmTargetPosition.ctl" = enum16{"Forward Cargo Floor Intake", "Forward Cargo Feeder Station", "Forward Cargo Low", "Forward Cargo Middle", "Forward Cargo High", "Forward Cargo CargoShip", "Forward Hatch Floor Intake", "Forward Hatch Feeder Station", "Forward Hatch Low", "Forward Hatch Middle", "Forward Hatch High", "Forward Hatch CargoShip", "Reverse Cargo Floor Intake", "Reverse Cargo Feeder Station", "Reverse Cargo Low", "Reverse Cargo Middle", "Reverse Cargo High", "Reverse Cargo CargoShip", "Reverse Hatch Floor Intake", "Reverse Hatch Feeder Station", "Reverse Hatch Low", "Reverse Hatch Middle", "Reverse Hatch High", "Reverse Hatch CargoShip", "Hold"}
  T12 = typedef "ArmPlanResponse.ctl" = cluster{"ShoulderTrajectory":T13[], "ExtendTrajectory":T13[], "PlanTime (ms)":u32, "Execute":bool, "WristTrajectory":T13[]}
  T13 = typedef "ArgosLib.lvlib/TrajectoryPoint.ctl" = cluster{"Position ":dbl, "Velocity ":dbl, "Time (ms)":T14, "Last Point":bool}
  T14 = typedef "CTRE_Phoenix_MotorControl_TrajectoryPointTimeDur.ctl" = i32
  T15 = typedef "Config_Robot.ctl" = cluster{"Motors":cluster{"DriveRightPrimary":T16, "DriveRightSecondary":T16, "DriveLeftPrimary":T16, "DriveLeftSecondary":T16, "RearClimb":T16, "Front Climb":T16, "Climb Drive":T16, "Shoulder1":T16, "Shoulder2":T16, "Wrist":T16, "Extension":T16, "CargoIntake":T16, "Intake2":T16}, "Sensors":cluster{"IMU":T20, "HomingButton":T22, "HomingLED_Green":T22, "HomingLED_Yellow":T22, "HomingLED_Red":T22}, "PID":cluster{"FrontClimb":T23, "RearClimb":T23, "ArmShoulder":T23, "ArmExtend":T23, "ArmWrist":T23}, "Solenoids":cluster{" Shifter":T24, "Hatch Grip":T24, "Hatch Extend":T24, "Manipulator Slide":T24, "Hatch Floor Intake":T24}, "Enable Compressor":bool, "MotionMagic":cluster{"FrontClimbExtend":T26, "RearClimbExtend":T26, "FrontClimbRetract":T26, "RearClimbRetract":T26}, "RobotDimensions":T3, "Arm Home Position":T27, "Climb Home Position":cluster{"Back Climb":dbl, "Front Climb":dbl}, "Climb Positions":T28}
  T16 = typedef "ArgosLib.lvlib/Config_Motor.ctl" = cluster{"CAN Address":u8, "Invert":bool, "InvertSensor":bool, "Unit Conversion Factor":dbl, "Brake Mode":T17, "Reverse Limt Switch Mode":T18, "Forward Limt Swith Mode":T18, "PWM Channel":T7, "Motor Controller Type":T19, "Peak Current (A)":i32, "Continuous Current (A)":i32, "Peak Duration (ms)":i32, "Current Limit Enable":bool}
  T17 = typedef "CTRE_Phoenix_MotorControl_NeutralMode.ctl" = enum8{"EEPROMSetting", "Override to Coast", "Override to Brake"}
  T18 = typedef "CTRE_Phoenix_MotorControl_LimitSwitchNormal.ctl" = enum16{"Normally Open", "Normally Closed", "Disabled"}
  T19 = typedef "ArgosLib.lvlib/Config_MotorCtrlType.ctl" = enum16{"Disabled", "Talon SRX", "Talon SR", "Venom"}
  T20 = typedef "ArgosLib.lvlib/Config_IMU.ctl" = cluster{"Yaw Axis":enum16{"X", "Y", "Z"}, "SPI Bus":T21, "AHRS Algorithm":enum16{"Complementary", "Madgwick"}, "Calibration Time (s)":dbl, "Calibrate On Open":bool}
  T21 = typedef "spi_bus.ctl" = enum16{"SPI On-Board, CS0", "SPI On-Board, CS1", "SPI On-Board, CS2", "SPI On-Board, CS3", "SPI MXP", "Invalid"}
  T22 = typedef "ArgosLib.lvlib/Config_DigitalIO.ctl" = cluster{"DIOChannel":T9, "Active Low":bool}
  T23 = typedef "ArgosLib.lvlib/Config_PIDParams.ctl" = cluster{"P":dbl, "I":dbl, "D":dbl, "F":dbl, "IZone":dbl}
  T24 = typedef "ArgosLib.lvlib/Config_SingleSolenoid.ctl" = cluster{"SolenoidChannel":T25, "Invert":bool}
  T25 = typedef "WPI_SolenoidChannel.ctl" = enum8{"Solenoid 0", "Solenoid 1", "Solenoid 2", "Solenoid 3", "Solenoid 4", "Solenoid 5", "Solenoid 6", "Solenoid 7", "Invalid"}
  T26 = typedef "Config_MotionMagicParams.ctl" = cluster{"CruiseVelocity":i32, "Acceleration":i32}
  T27 = typedef "ArmCoordinate.ctl" = cluster{"Radius (in)":dbl, "ShoulderAngle (rad)":dbl, "WristAngle (rad)":dbl}
  T28 = typedef "ClimberPositionHeights.ctl" = cluster{"Retract":dbl, "Level 2":dbl, "Level 3":dbl}
  T29 = typedef "ArgosLib.lvlib/MotionProfileGeneratorParams.ctl" = cluster{"Trajectory Point Interval (ms)":T14, "Maximum Travel Speed (units/s)":dbl, "Velocity Ramp Time (ms)":dbl, "Acceleration Ramp Time (ms)":dbl}
  T30 = typedef "ArgosLib.lvlib/Polygon2D.ctl" = T31[]
  T31 = typedef "ArgosLib.lvlib/Point2D.ctl" = cluster{"X (in)":dbl, "Y (in)":dbl}
  T32 = typedef "GamePiecePosition.ctl" = cluster{"Hatch Forward":T33, "Hatch Reverse":T33, "Cargo Forward":T33, "Cargo Reverse":T33, "Hold":T1}
  T33 = typedef "ArmPositions.ctl" = cluster{"FeederStation":T1, "Low":T1, "Mid":T1, "High":T1, "FloorIntake":T1, "CargoShip":T1}
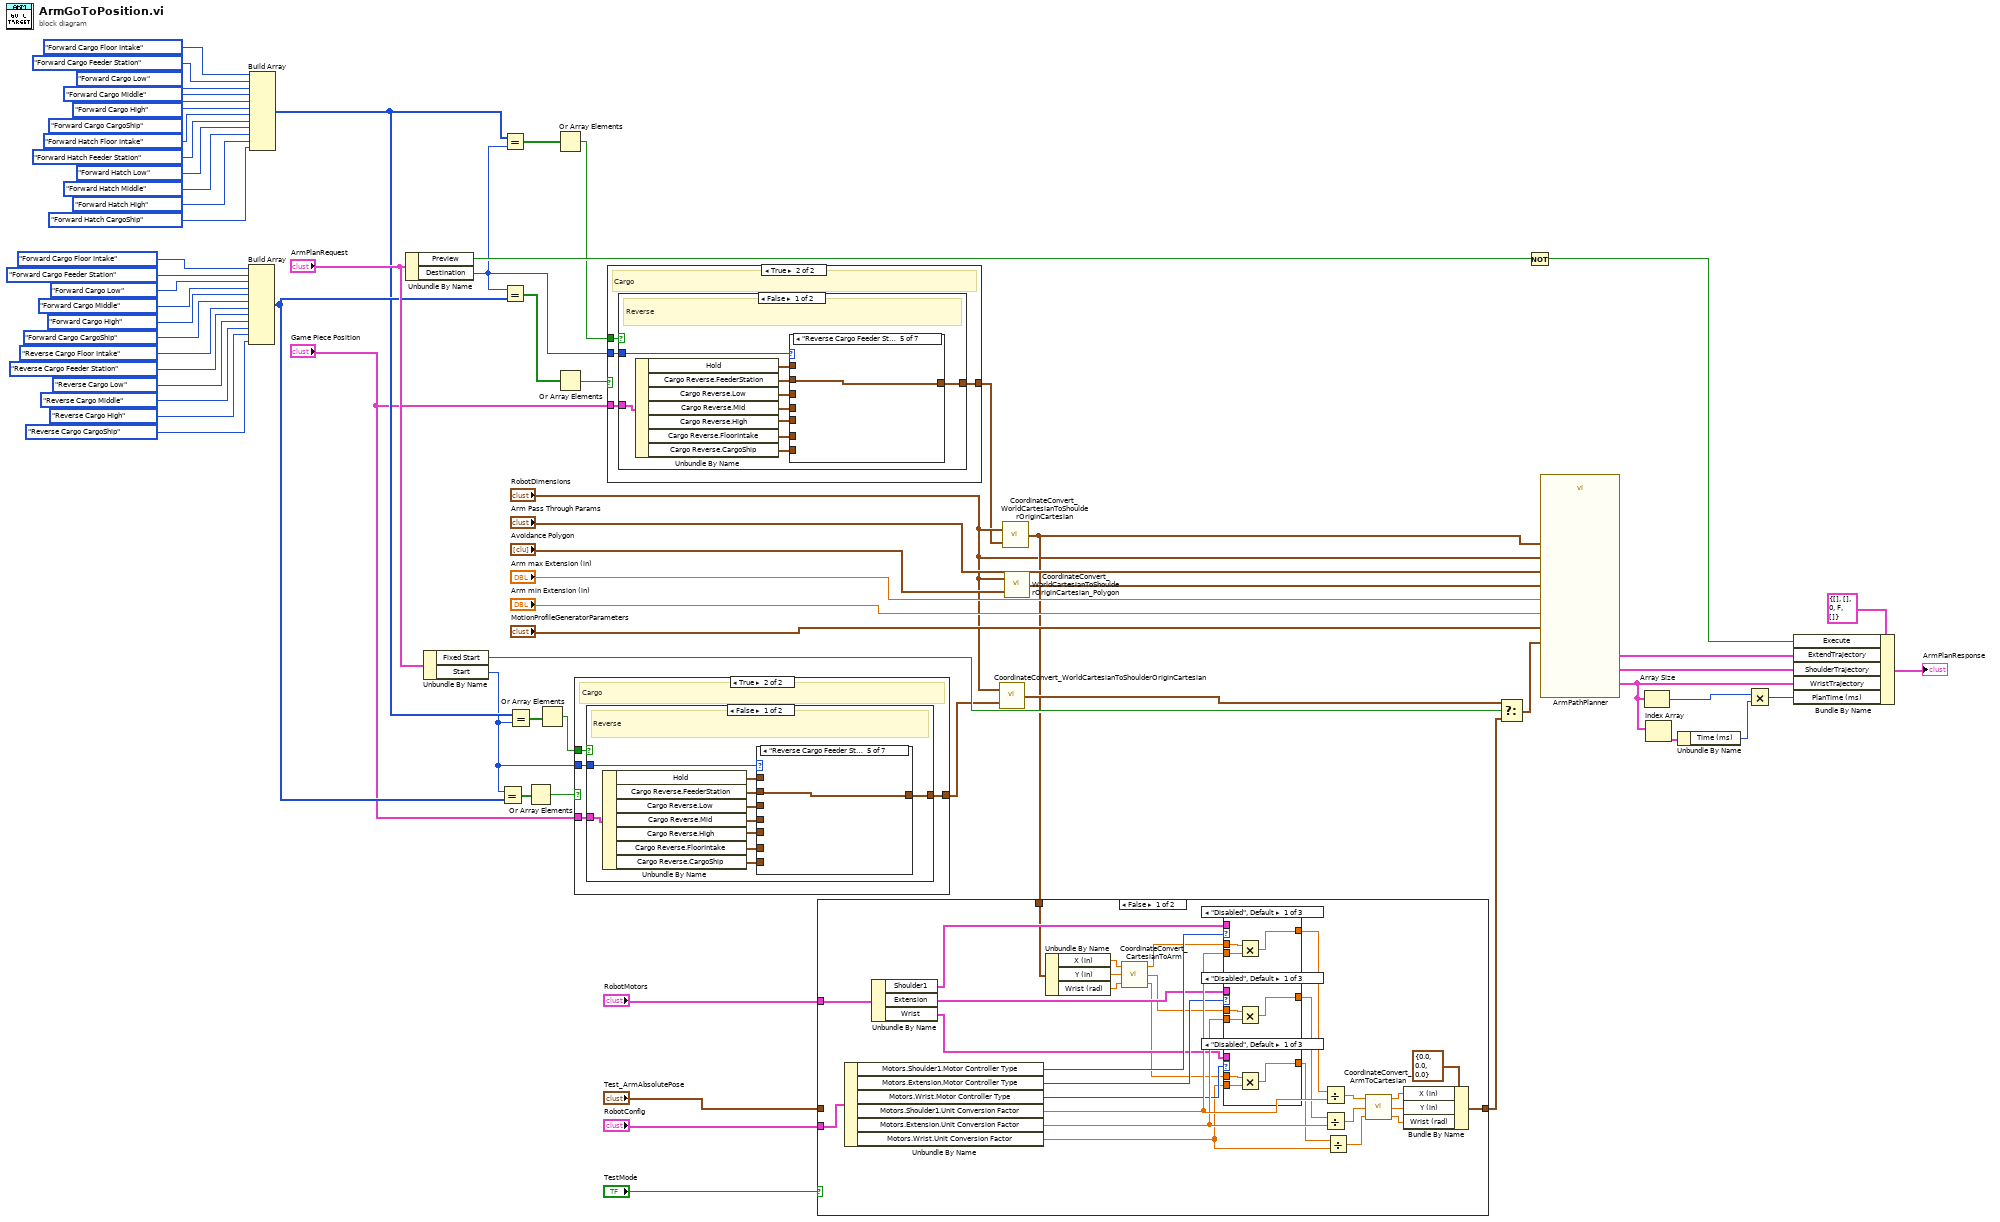
[diagram p0: block diagram]
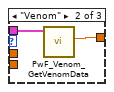
[diagram p2: hidden frame]
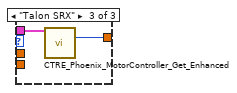
[diagram p3: hidden frame]
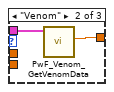
[diagram p4: hidden frame]
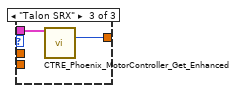
[diagram p5: hidden frame]
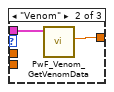
[diagram p6: hidden frame]
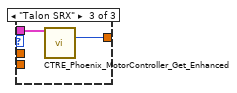
[diagram p7: hidden frame]
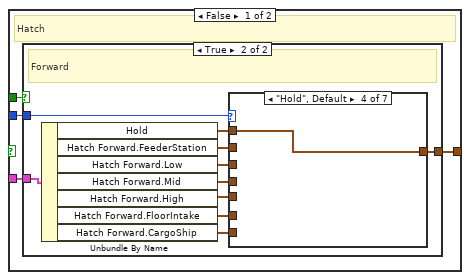
[diagram p9: hidden frame]
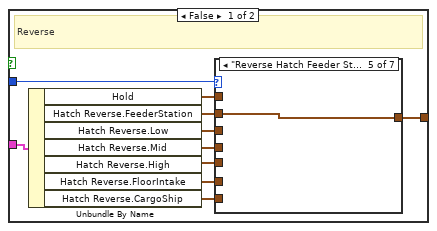
[diagram p10: hidden frame]
diagram:
  n1 = Build Array(ArmTargetPosition."Forward Cargo Floor Intake" ("Destination"), ArmTargetPosition."Forward Cargo Feeder Station" ("Destination"), ArmTargetPosition."Forward Cargo Low" ("Destination"), ArmTargetPosition."Forward Cargo Middle" ("Destination"), ArmTargetPosition."Forward Cargo High" ("Destination"), ArmTargetPosition."Forward Cargo CargoShip" ("Destination"), ArmTargetPosition."Reverse Cargo Floor Intake" ("Destination"), ArmTargetPosition."Reverse Cargo Feeder Station" ("Destination"), ArmTargetPosition."Reverse Cargo Low" ("Destination"), ArmTargetPosition."Reverse Cargo Middle" ("Destination"), ArmTargetPosition."Reverse Cargo High" ("Destination"), ArmTargetPosition."Reverse Cargo CargoShip" ("Destination")) -> (w21:T11[])
  n2 = Build Array(ArmTargetPosition."Forward Cargo Floor Intake" ("Destination"), ArmTargetPosition."Forward Cargo Feeder Station" ("Destination"), ArmTargetPosition."Forward Cargo Low" ("Destination"), ArmTargetPosition."Forward Cargo Middle" ("Destination"), ArmTargetPosition."Forward Cargo High" ("Destination"), ArmTargetPosition."Forward Cargo CargoShip" ("Destination"), ArmTargetPosition."Forward Hatch Floor Intake" ("Destination"), ArmTargetPosition."Forward Hatch Feeder Station" ("Destination"), ArmTargetPosition."Forward Hatch Low" ("Destination"), ArmTargetPosition."Forward Hatch Middle" ("Destination"), ArmTargetPosition."Forward Hatch High" ("Destination"), ArmTargetPosition."Forward Hatch CargoShip" ("Destination")) -> (w18:T11[])
  n3 = Unbundle By Name("ArmPlanRequest") -> ("Preview"=w56:bool, "Destination"=w22:T11)
  n4 = Unbundle By Name("ArmPlanRequest") -> ("Fixed Start"=w50:bool, "Start"=w9:T11)
  n5 = Equal?(x=w9, y=w21) -> (x = y?=w20:bool[])
  n6 = Equal?(x=w18, y=w22) -> (x = y?=w24:bool[])
  n7 = Equal?(x=w22, y=w21) -> (x = y?=w36:bool[])
  n8 = Equal?(x=w18, y=w9) -> (x = y?=w19:bool[])
  n9 = Or Array Elements(Boolean array=w20) -> (logical OR=w8:bool)
  n10 = Or Array Elements(Boolean array=w19) -> (logical OR=w10:bool)
  n11 = Or Array Elements(Boolean array=w24) -> (logical OR=w23:bool)
  n12 = Or Array Elements(Boolean array=w36) -> (logical OR=w35:bool)
  n13 = case shown="True" w8 {
    tunnel: [w68 w106] -> w6
    tunnel: "Game Piece Position" -> [w69 w107]
    tunnel: w10 -> [w71 w109]
    tunnel: w9 -> [w70 w108]
    frame False {
      # "Hatch"
      n14 = case shown="True" w71 {
        tunnel: w70 -> [w81 w98]
        tunnel: w69 -> [w80 w97]
        tunnel: [w74 w91] -> w68
        frame False {
          # "Reverse"
          n15 = Unbundle By Name(w80) -> ("Hold"=w79:T1, "Hatch Reverse.FeederStation"=w78:T1, "Hatch Reverse.Low"=w77:T1, "Hatch Reverse.Mid"=w76:T1, "Hatch Reverse.High"=w75:T1, "Hatch Reverse.FloorIntake"=w73:T1, "Hatch Reverse.CargoShip"=w72:T1)
          n16 = case shown="\"Reverse Hatch Feeder Station\"" w81 {
            tunnel: w79 -> [_ _ _ w85 _ _ _]
            tunnel: w78 -> [_ _ _ _ w86 _ _]
            tunnel: w77 -> [_ _ _ _ _ w87 _]
            tunnel: w76 -> [_ _ _ _ _ _ w88]
            tunnel: w75 -> [w82 _ _ _ _ _ _]
            tunnel: [w82 w83 w84 w85 w86 w87 w88] -> w74
            tunnel: w73 -> [_ w83 _ _ _ _ _]
            tunnel: w72 -> [_ _ w84 _ _ _ _]
            frame "Reverse Hatch High" {
            }
            frame "Reverse Hatch Floor Intake" {
            }
            frame "Reverse Hatch CargoShip" {
            }
            frame "Hold", Default {
            }
            frame "Reverse Hatch Feeder Station" {
            }
            frame "Reverse Hatch Low" {
            }
            frame "Reverse Hatch Middle" {
            }
          }
        }
        frame True {
          # "Forward"
          n17 = Unbundle By Name(w97) -> ("Hold"=w96:T1, "Hatch Forward.FeederStation"=w95:T1, "Hatch Forward.Low"=w94:T1, "Hatch Forward.Mid"=w93:T1, "Hatch Forward.High"=w92:T1, "Hatch Forward.FloorIntake"=w90:T1, "Hatch Forward.CargoShip"=w89:T1)
          n18 = case shown="\"Hold\", Default" w98 {
            tunnel: w96 -> [_ _ _ w102 _ _ _]
            tunnel: w95 -> [_ _ _ _ w103 _ _]
            tunnel: w94 -> [_ _ _ _ _ w104 _]
            tunnel: w93 -> [_ _ _ _ _ _ w105]
            tunnel: w92 -> [w99 _ _ _ _ _ _]
            tunnel: [w99 w100 w101 w102 w103 w104 w105] -> w91
            tunnel: w90 -> [_ w100 _ _ _ _ _]
            tunnel: w89 -> [_ _ w101 _ _ _ _]
            frame "Forward Hatch High" {
            }
            frame "Forward Hatch Floor Intake" {
            }
            frame "Forward Hatch CargoShip" {
            }
            frame "Hold", Default {
            }
            frame "Forward Hatch Feeder Station" {
            }
            frame "Forward Hatch Low" {
            }
            frame "Forward Hatch Middle" {
            }
          }
        }
      }
    }
    frame True {
      # "Cargo"
      n19 = case shown="False" w109 {
        tunnel: w108 -> [w119 w136]
        tunnel: w107 -> [w118 w135]
        tunnel: [w112 w129] -> w106
        frame False {
          # "Reverse"
          n20 = Unbundle By Name(w118) -> ("Hold"=w117:T1, "Cargo Reverse.FeederStation"=w116:T1, "Cargo Reverse.Low"=w115:T1, "Cargo Reverse.Mid"=w114:T1, "Cargo Reverse.High"=w113:T1, "Cargo Reverse.FloorIntake"=w111:T1, "Cargo Reverse.CargoShip"=w110:T1)
          n21 = case shown="\"Reverse Cargo Feeder Station\"" w119 {
            tunnel: w117 -> [_ _ _ w123 _ _ _]
            tunnel: w116 -> [_ _ _ _ w124 _ _]
            tunnel: w115 -> [_ _ _ _ _ w125 _]
            tunnel: w114 -> [_ _ _ _ _ _ w126]
            tunnel: w113 -> [w120 _ _ _ _ _ _]
            tunnel: [w120 w121 w122 w123 w124 w125 w126] -> w112
            tunnel: w111 -> [_ w121 _ _ _ _ _]
            tunnel: w110 -> [_ _ w122 _ _ _ _]
            frame "Reverse Cargo High" {
            }
            frame "Reverse Cargo Floor Intake" {
            }
            frame "Reverse Cargo CargoShip" {
            }
            frame "Hold", Default {
            }
            frame "Reverse Cargo Feeder Station" {
            }
            frame "Reverse Cargo Low" {
            }
            frame "Reverse Cargo Middle" {
            }
          }
        }
        frame True {
          # "Forward"
          n22 = Unbundle By Name(w135) -> ("Hold"=w134:T1, "Cargo Forward.FeederStation"=w133:T1, "Cargo Forward.Low"=w132:T1, "Cargo Forward.Mid"=w131:T1, "Cargo Forward.High"=w130:T1, "Cargo Forward.FloorIntake"=w128:T1, "Cargo Forward.CargoShip"=w127:T1)
          n23 = case shown="\"Hold\", Default" w136 {
            tunnel: w134 -> [_ _ _ w140 _ _ _]
            tunnel: w133 -> [_ _ _ _ w141 _ _]
            tunnel: w132 -> [_ _ _ _ _ w142 _]
            tunnel: w131 -> [_ _ _ _ _ _ w143]
            tunnel: w130 -> [w137 _ _ _ _ _ _]
            tunnel: [w137 w138 w139 w140 w141 w142 w143] -> w129
            tunnel: w128 -> [_ w138 _ _ _ _ _]
            tunnel: w127 -> [_ _ w139 _ _ _ _]
            frame "Forward Cargo High" {
            }
            frame "Forward Cargo Floor Intake" {
            }
            frame "Forward Cargo CargoShip" {
            }
            frame "Hold", Default {
            }
            frame "Forward Cargo Feeder Station" {
            }
            frame "Forward Cargo Low" {
            }
            frame "Forward Cargo Middle" {
            }
          }
        }
      }
    }
  }
  n24 = case shown="True" w35 {
    tunnel: [w144 w182] -> w1
    tunnel: "Game Piece Position" -> [w145 w183]
    tunnel: w23 -> [w147 w185]
    tunnel: w22 -> [w146 w184]
    frame False {
      # "Hatch"
      n25 = case shown="True" w147 {
        tunnel: w146 -> [w157 w174]
        tunnel: w145 -> [w156 w173]
        tunnel: [w150 w167] -> w144
        frame False {
          # "Reverse"
          n26 = Unbundle By Name(w156) -> ("Hold"=w155:T1, "Hatch Reverse.FeederStation"=w154:T1, "Hatch Reverse.Low"=w153:T1, "Hatch Reverse.Mid"=w152:T1, "Hatch Reverse.High"=w151:T1, "Hatch Reverse.FloorIntake"=w149:T1, "Hatch Reverse.CargoShip"=w148:T1)
          n27 = case shown="\"Reverse Hatch Feeder Station\"" w157 {
            tunnel: w155 -> [_ _ _ w161 _ _ _]
            tunnel: w154 -> [_ _ _ _ w162 _ _]
            tunnel: w153 -> [_ _ _ _ _ w163 _]
            tunnel: w152 -> [_ _ _ _ _ _ w164]
            tunnel: w151 -> [w158 _ _ _ _ _ _]
            tunnel: [w158 w159 w160 w161 w162 w163 w164] -> w150
            tunnel: w149 -> [_ w159 _ _ _ _ _]
            tunnel: w148 -> [_ _ w160 _ _ _ _]
            frame "Reverse Hatch High" {
            }
            frame "Reverse Hatch Floor Intake" {
            }
            frame "Reverse Hatch CargoShip" {
            }
            frame "Hold", Default {
            }
            frame "Reverse Hatch Feeder Station" {
            }
            frame "Reverse Hatch Low" {
            }
            frame "Reverse Hatch Middle" {
            }
          }
        }
        frame True {
          # "Forward"
          n28 = Unbundle By Name(w173) -> ("Hold"=w172:T1, "Hatch Forward.FeederStation"=w171:T1, "Hatch Forward.Low"=w170:T1, "Hatch Forward.Mid"=w169:T1, "Hatch Forward.High"=w168:T1, "Hatch Forward.FloorIntake"=w166:T1, "Hatch Forward.CargoShip"=w165:T1)
          n29 = case shown="\"Hold\", Default" w174 {
            tunnel: w172 -> [_ _ _ w178 _ _ _]
            tunnel: w171 -> [_ _ _ _ w179 _ _]
            tunnel: w170 -> [_ _ _ _ _ w180 _]
            tunnel: w169 -> [_ _ _ _ _ _ w181]
            tunnel: w168 -> [w175 _ _ _ _ _ _]
            tunnel: [w175 w176 w177 w178 w179 w180 w181] -> w167
            tunnel: w166 -> [_ w176 _ _ _ _ _]
            tunnel: w165 -> [_ _ w177 _ _ _ _]
            frame "Forward Hatch High" {
            }
            frame "Forward Hatch Floor Intake" {
            }
            frame "Forward Hatch CargoShip" {
            }
            frame "Hold", Default {
            }
            frame "Forward Hatch Feeder Station" {
            }
            frame "Forward Hatch Low" {
            }
            frame "Forward Hatch Middle" {
            }
          }
        }
      }
    }
    frame True {
      # "Cargo"
      n30 = case shown="False" w185 {
        tunnel: w184 -> [w195 w212]
        tunnel: w183 -> [w194 w211]
        tunnel: [w188 w205] -> w182
        frame False {
          # "Reverse"
          n31 = Unbundle By Name(w194) -> ("Hold"=w193:T1, "Cargo Reverse.FeederStation"=w192:T1, "Cargo Reverse.Low"=w191:T1, "Cargo Reverse.Mid"=w190:T1, "Cargo Reverse.High"=w189:T1, "Cargo Reverse.FloorIntake"=w187:T1, "Cargo Reverse.CargoShip"=w186:T1)
          n32 = case shown="\"Reverse Cargo Feeder Station\"" w195 {
            tunnel: w193 -> [_ _ _ w199 _ _ _]
            tunnel: w192 -> [_ _ _ _ w200 _ _]
            tunnel: w191 -> [_ _ _ _ _ w201 _]
            tunnel: w190 -> [_ _ _ _ _ _ w202]
            tunnel: w189 -> [w196 _ _ _ _ _ _]
            tunnel: [w196 w197 w198 w199 w200 w201 w202] -> w188
            tunnel: w187 -> [_ w197 _ _ _ _ _]
            tunnel: w186 -> [_ _ w198 _ _ _ _]
            frame "Reverse Cargo High" {
            }
            frame "Reverse Cargo Floor Intake" {
            }
            frame "Reverse Cargo CargoShip" {
            }
            frame "Hold", Default {
            }
            frame "Reverse Cargo Feeder Station" {
            }
            frame "Reverse Cargo Low" {
            }
            frame "Reverse Cargo Middle" {
            }
          }
        }
        frame True {
          # "Forward"
          n33 = Unbundle By Name(w211) -> ("Hold"=w210:T1, "Cargo Forward.FeederStation"=w209:T1, "Cargo Forward.Low"=w208:T1, "Cargo Forward.Mid"=w207:T1, "Cargo Forward.High"=w206:T1, "Cargo Forward.FloorIntake"=w204:T1, "Cargo Forward.CargoShip"=w203:T1)
          n34 = case shown="\"Hold\", Default" w212 {
            tunnel: w210 -> [_ _ _ w216 _ _ _]
            tunnel: w209 -> [_ _ _ _ w217 _ _]
            tunnel: w208 -> [_ _ _ _ _ w218 _]
            tunnel: w207 -> [_ _ _ _ _ _ w219]
            tunnel: w206 -> [w213 _ _ _ _ _ _]
            tunnel: [w213 w214 w215 w216 w217 w218 w219] -> w205
            tunnel: w204 -> [_ w214 _ _ _ _ _]
            tunnel: w203 -> [_ _ w215 _ _ _ _]
            frame "Forward Cargo High" {
            }
            frame "Forward Cargo Floor Intake" {
            }
            frame "Forward Cargo CargoShip" {
            }
            frame "Hold", Default {
            }
            frame "Forward Cargo Feeder Station" {
            }
            frame "Forward Cargo Low" {
            }
            frame "Forward Cargo Middle" {
            }
          }
        }
      }
    }
  }
  n35 = call "CoordinateConvert_WorldCartesianToShoulderOriginCartesian.vi"("ArmPositionIn"=w6, "RobotDimensions"="RobotDimensions") -> ("ArmPositionRelativeToShoulder"=w16:T1)
  n36 = call "CoordinateConvert_WorldCartesianToShoulderOriginCartesian.vi"("ArmPositionIn"=w1, "RobotDimensions"="RobotDimensions") -> ("ArmPositionRelativeToShoulder"=w3:T1)
  n37 = case shown="False" "TestMode" {
    tunnel: "RobotConfig" -> [w248 _]
    tunnel: [w241 w270] -> w52
    tunnel: "RobotMotors" -> [w238 _]
    tunnel: "Test_ArmAbsolutePose" -> [_ w270]
    tunnel: w3 -> [w235 _]
    frame False {
      n38 = Unbundle By Name(w248) -> ("Motors.Shoulder1.Motor Controller Type"=w236:T19, "Motors.Extension.Motor Controller Type"=w227:T19, "Motors.Wrist.Motor Controller Type"=w224:T19, "Motors.Shoulder1.Unit Conversion Factor"=w230:dbl, "Motors.Extension.Unit Conversion Factor"=w225:dbl, "Motors.Wrist.Unit Conversion Factor"=w221:dbl)
      n39 = Unbundle By Name(w238) -> ("Shoulder1"=w237:T5, "Extension"=w228:T5, "Wrist"=w223:T5)
      n40 = Unbundle By Name(w235) -> ("X (in)"=w234:dbl, "Y (in)"=w233:dbl, "Wrist (rad)"=w232:dbl)
      n41 = call "CoordinateConvert_CartesianToArm.vi"("Wrist (rad)"=w232, "Y (in)"=w233, "X (in)"=w234) -> ("Wrist Angle (rad)"=w220:dbl, "Radius (in)"=w226:dbl, "Shoulder Angle (rad)"=w231:dbl)
      n42 = case shown="\"Disabled\", Default" w236 {
        tunnel: [w263 w267 w269] -> w247
        tunnel: w237 -> [_ w266 w268]
        tunnel: w231 -> [w264 _ _]
        tunnel: w230 -> [w265 _ _]
        frame "Disabled", Default {
          n43 = Multiply(x=w264, y=w265) -> (x*y=w263:dbl)
        }
        frame "Venom" {
          n44 = call-poly <vilib>:"PwF_Venom_GetVenomData.vi"("PwFVenomDevRefIn"=w266) -> ("Position"=w267:dbl)  [unwired: 8 in, 2 out]
        }
        frame "Talon SRX" {
          n45 = call-poly <vilib>:"CTRE_Phoenix_MotorController_Get_Enhanced.vi"("PhoenixMotorControlDevRef"=w268) -> ("Position (Raw Sensor Units)"=w269:i32)  [unwired: 11 in, 3 out]
        }
      }
      n46 = case shown="\"Disabled\", Default" w227 {
        tunnel: [w256 w260 w262] -> w229
        tunnel: w228 -> [_ w259 w261]
        tunnel: w226 -> [w257 _ _]
        tunnel: w225 -> [w258 _ _]
        frame "Disabled", Default {
          n47 = Multiply(x=w257, y=w258) -> (x*y=w256:dbl)
        }
        frame "Venom" {
          n48 = call-poly <vilib>:"PwF_Venom_GetVenomData.vi"("PwFVenomDevRefIn"=w259) -> ("Position"=w260:dbl)  [unwired: 8 in, 2 out]
        }
        frame "Talon SRX" {
          n49 = call-poly <vilib>:"CTRE_Phoenix_MotorController_Get_Enhanced.vi"("PhoenixMotorControlDevRef"=w261) -> ("Position (Raw Sensor Units)"=w262:i32)  [unwired: 11 in, 3 out]
        }
      }
      n50 = case shown="\"Disabled\", Default" w224 {
        tunnel: [w249 w253 w255] -> w222
        tunnel: w223 -> [_ w252 w254]
        tunnel: w220 -> [w250 _ _]
        tunnel: w221 -> [w251 _ _]
        frame "Disabled", Default {
          n51 = Multiply(x=w250, y=w251) -> (x*y=w249:dbl)
        }
        frame "Venom" {
          n52 = call-poly <vilib>:"PwF_Venom_GetVenomData.vi"("PwFVenomDevRefIn"=w252) -> ("Position"=w253:dbl)  [unwired: 8 in, 2 out]
        }
        frame "Talon SRX" {
          n53 = call-poly <vilib>:"CTRE_Phoenix_MotorController_Get_Enhanced.vi"("PhoenixMotorControlDevRef"=w254) -> ("Position (Raw Sensor Units)"=w255:i32)  [unwired: 11 in, 3 out]
        }
      }
      n54 = Divide(x=w247, y=w230) -> (x/y=w246:dbl)
      n55 = Divide(x=w229, y=w225) -> (x/y=w245:dbl)
      n56 = Divide(x=w222, y=w221) -> (x/y=w240:dbl)
      n57 = call "CoordinateConvert_ArmToCartesian.vi"("Wrist Angle (rad)"=w240, "Radius (in)"=w245, "Shoulder Angle (rad)"=w246) -> ("Wrist (rad)"=w239:dbl, "Y (in)"=w242:dbl, "X (in)"=w243:dbl)
      n58 = Bundle By Name(cluster=T1 {"X (in)"=0.0, "Y (in)"=0.0, "Wrist (rad)"=0.0} ("ArmAbsolutePose"), "X (in)"=w243, "Y (in)"=w242, "Wrist (rad)"=w239) -> (w241:T1)
    }
    frame True {
    }
  }
  n59 = call "CoordinateConvert_WorldCartesianToShoulderOriginCartesian_Polygon.vi"("ArmPositionIn"="Avoidance Polygon", "RobotDimensions"="RobotDimensions") -> ("ArmPositionRelativeToShoulder"=w15:T30)
  n60 = Select(t=w16, s=w50, f=w52) -> (s? t:f=w51:T1)
  n61 = Not(x=w56) -> (.not. x?=w54:bool)
  n62 = call "ArmPathPlanner.vi"("StartPoint"=w51, "EndPoint"=w3, "MinArmLength"="Arm min Extension (in)", "MaxArmLength"="Arm max Extension (in)", "AvoidancePolygon"=w15, "RobotDimensions"="RobotDimensions", "MotionProfileGeneratorParameters"="MotionProfileGeneratorParameters", "Arm Pass Through Params"="Arm Pass Through Params") -> ("ShoulderPath"=w60:T13[], "ExtendPath"=w61:T13[], "WristPath"=w47:T13[])  [unwired: 7 in, 2 out]
  n63 = Array Size(array=w47) -> (size(s)=w58:i32)
  n64 = Index Array(array=w47) -> (element=w59:T13)  [unwired: 1 in]
  n65 = Unbundle By Name(w59) -> ("Time (ms)"=w57:T14)
  n66 = Multiply(x=w58, y=w57) -> (x*y=w48:T14)
  n67 = Bundle By Name(cluster=T12 {"ShoulderTrajectory"=[], "ExtendTrajectory"=[], "PlanTime (ms)"=0, "Execute"=FALSE, "WristTrajectory"=[]} ("ArmPlanResponse"), "Execute"=w54, "ExtendTrajectory"=w61, "ShoulderTrajectory"=w60, "WristTrajectory"=w47, "PlanTime (ms)"=w48) -> (→"ArmPlanResponse":T12)
